vi "MoveAbsolute.vi"(8 "error in (no error)":errorcluster, 11 "XYStage in":refnum<class "XYStage.lvclass">) -> (0 "error out":errorcluster, 3 "XYStage out":refnum<class "XYStage.lvclass">)   [LabVIEW 2017, in "XYStage.lvclass"]
uses:
  XYStage.lvclass
  Typedefs/Coordinates.Units--Cluster.ctl
panel:
  in  "Units":T1
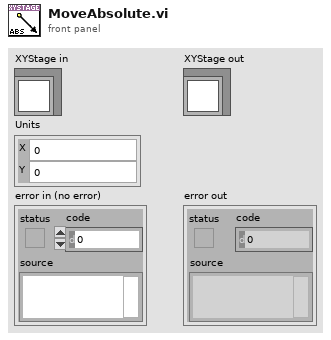
[diagram p1: front panel]
types:
  T1 = typedef "XYStage.lvclass/Coordinates.Units--Cluster.ctl" = cluster{"X":dbl, "Y":dbl}
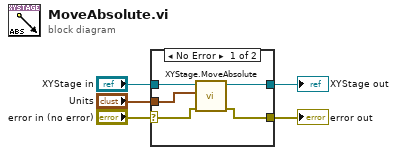
[diagram p0: block diagram]
diagram:
  n1 = case shown="No Error" "error in (no error)" {
    selector: "error in (no error)" -> [w9 w12]
    tunnel: [w8 w12] -> w4
    tunnel: [w7 w11] -> w2
    tunnel: "XYStage in" -> [w10 w11]
    tunnel: "Units" -> [w6 _]
    frame No Error {
      n2 = call-dynamic "XYStage.MoveAbsolute.vi"("error in (no error)"=w9, "Units"=w6, "XYStage in"=w10) -> ("error out"=w8:errorcluster, "XYStage out"=w7:refnum<class "XYStage.lvclass">)  [unwired: 7 in]
    }
    frame Error {
    }
  }
  "error out" <- w4
  "XYStage out" <- w2
